vi "update.vi"(8 "error in (no error)":errorcluster, 10 "adapter executability":T1={"instrument"=TRUE, "trajectory"=TRUE, "scanHead"=TRUE, "DAQ"=TRUE, "imageAssembler"=TRUE, "dataCollection"=TRUE, "display"=TRUE, "analyser"=TRUE, "stimulator"=TRUE}, 11 "ScanModeDL090923Scaffold in":refnum<class "ImagingModeDL090923Scaffold.lvclass">) -> (0 "error out":errorcluster, 3 "ScanModeDL090923Scaffold out":refnum<class "ImagingModeDL090923Scaffold.lvclass">)   [LabVIEW 2010, in "ImagingModeDL090923Scaffold.lvclass"]
uses:
  ImagingModeDL090923Scaffold.lvclass
  adapter_executability_cluster.ctl
  Instrument/GenericInstrument/GenericInstrument/GenericInstrument.lvclass
  Trajectory/GenericTrajectory/GenericTrajectory/GenericTrajectory.lvclass
  ScanHead/GenericScanHead/GenericScanHead/GenericScanHead.lvclass
  Stimulator/GenericStimulator/GenericStimulator/GenericStimulator.lvclass
  Analyser/GenericAnalyser/GenericAnalyser/GenericAnalyser.lvclass
  DataCollection/GenericDataCollection/GenericDataCollection/GenericDataCollection.lvclass
  Display/GenericDisplay/GenericDisplay/GenericDisplay.lvclass
  ImageAssembler/GenericImageAssembler/GenericImageAssembler/GenericImageAssembler.lvclass
  DAQ/GenericDAQ/GenericDAQ/GenericDAQ.lvclass
  common/classes/GenericComponent/GenericComponent/GenericComponent.lvclass
  GenericImagingMode/GenericImagingMode/GenericImagingMode.lvclass
  Adapter/GenericAdapter/GenericAdapter/GenericAdapter.lvclass
  common/classes/ErrorController/ErrorController/class_data.vi
  common/classes/ErrorController/ErrorController/ErrorController.lvclass
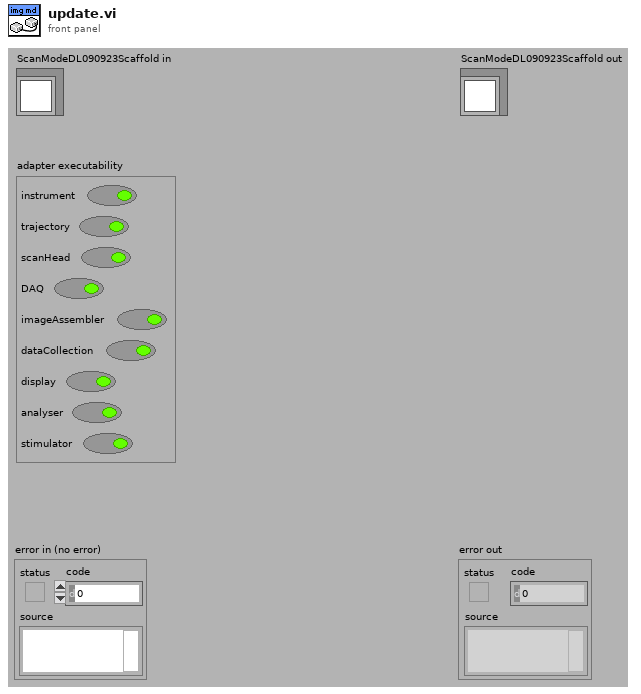
[diagram p1: front panel]
types:
  T1 = typedef "ImagingModeDL090923Scaffold.lvclass/adapter_executability_cluster.ctl" = cluster{"instrument":bool, "trajectory":bool, "scanHead":bool, "DAQ":bool, "imageAssembler":bool, "dataCollection":bool, "display":bool, "analyser":bool, "stimulator":bool}
  T2 = cluster{"[0]":refnum<class "GenericComponent.lvclass">, "[1]":refnum<class "GenericComponent.lvclass">, "[2]":refnum<class "GenericComponent.lvclass">, "[3]":refnum<class "GenericComponent.lvclass">, "[4]":refnum<class "GenericComponent.lvclass">, "[5]":refnum<class "GenericComponent.lvclass">, "[6]":refnum<class "GenericComponent.lvclass">, "[7]":refnum<class "GenericComponent.lvclass">, "[8]":refnum<class "GenericComponent.lvclass">}
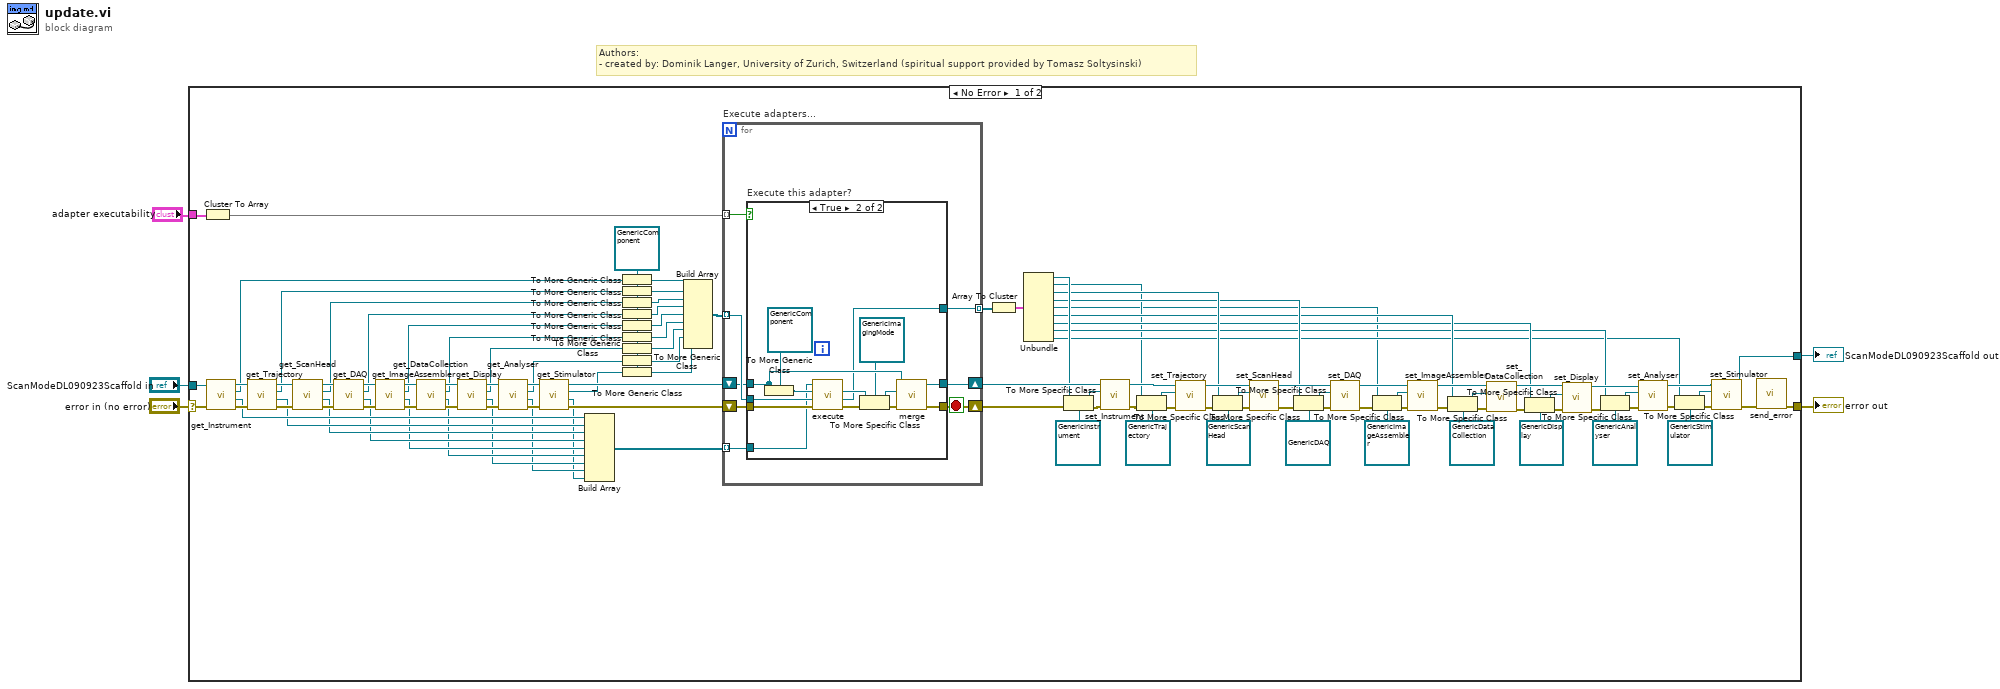
[diagram p0: block diagram]
diagram:
  # "Authors: \n- created by: Dominik Langer, University of Zurich, Switzerland (spiritual support provided by Tomasz Soltysinski)"
  n1 = case shown="No Error" "error in (no error)" {
    selector: "error in (no error)" -> [w76 w142]
    tunnel: [w27 w143] -> w2
    tunnel: "ScanModeDL090923Scaffold in" -> [w9 w143]
    tunnel: [w12 w142] -> w3
    tunnel: "adapter executability" -> [w7 _]
    frame No Error {
      w10 = refnum<class "GenericComponent.lvclass"> refnum ("GenericComponent.lvclass")
      n2 = Cluster To Array(cluster=w7) -> (array=w6:bool[])
      n3 = call-dynamic "get_Instrument.vi"("error in (no error)"=w76, "ScanModeDL090923Scaffold in"=w9) -> ("error out"=w84:errorcluster, "Instrument adapter"=w65:refnum<class "GenericAdapter.lvclass">, "Instrument"=w56:refnum<class "GenericInstrument.lvclass">, "ScanModeDL090923Scaffold out"=w74:refnum<class "ImagingModeDL090923Scaffold.lvclass">)  [unwired: 4 in, 2 out]
      n4 = call-dynamic "get_Trajectory.vi"("error in (no error)"=w84, "ScanModeDL090923Scaffold in"=w74) -> ("error out"=w83:errorcluster, "Trajectory adapter"=w64:refnum<class "GenericAdapter.lvclass">, "Trajectory"=w55:refnum<class "GenericTrajectory.lvclass">, "ScanModeDL090923Scaffold out"=w73:refnum<class "ImagingModeDL090923Scaffold.lvclass">)  [unwired: 2 in, 4 out]
      n5 = call-dynamic "get_ScanHead.vi"("error in (no error)"=w83, "ScanModeDL090923Scaffold in"=w73) -> ("error out"=w82:errorcluster, "ScanHead adapter"=w63:refnum<class "GenericAdapter.lvclass">, "ScanHead"=w54:refnum<class "GenericScanHead.lvclass">, "ScanModeDL090923Scaffold out"=w72:refnum<class "ImagingModeDL090923Scaffold.lvclass">)  [unwired: 4 in, 2 out]
      n6 = call-dynamic "get_DAQ.vi"("error in (no error)"=w82, "ScanModeDL090923Scaffold in"=w72) -> ("error out"=w81:errorcluster, "DAQ adapter"=w62:refnum<class "GenericAdapter.lvclass">, "DAQ"=w53:refnum<class "GenericDAQ.lvclass">, "ScanModeDL090923Scaffold out"=w71:refnum<class "ImagingModeDL090923Scaffold.lvclass">)  [unwired: 4 in, 2 out]
      n7 = call-dynamic "get_ImageAssembler.vi"("error in (no error)"=w81, "ScanModeDL090923Scaffold in"=w71) -> ("error out"=w80:errorcluster, "ImageAssembler adapter"=w61:refnum<class "GenericAdapter.lvclass">, "ImageAssembler"=w52:refnum<class "GenericImageAssembler.lvclass">, "ScanModeDL090923Scaffold out"=w70:refnum<class "ImagingModeDL090923Scaffold.lvclass">)  [unwired: 4 in, 2 out]
      n8 = call-dynamic "get_DataCollection.vi"("error in (no error)"=w80, "ScanModeDL090923Scaffold in"=w70) -> ("error out"=w79:errorcluster, "DataCollection adapter"=w60:refnum<class "GenericAdapter.lvclass">, "DataCollection"=w51:refnum<class "GenericDataCollection.lvclass">, "ScanModeDL090923Scaffold out"=w69:refnum<class "ImagingModeDL090923Scaffold.lvclass">)  [unwired: 4 in, 2 out]
      n9 = call-dynamic "get_Display.vi"("error in (no error)"=w79, "ScanModeDL090923Scaffold in"=w69) -> ("error out"=w78:errorcluster, "Display adapter"=w59:refnum<class "GenericAdapter.lvclass">, "Display"=w50:refnum<class "GenericDisplay.lvclass">, "ScanModeDL090923Scaffold out"=w68:refnum<class "ImagingModeDL090923Scaffold.lvclass">)  [unwired: 4 in, 2 out]
      n10 = call-dynamic "get_Analyser.vi"("error in (no error)"=w78, "ScanModeDL090923Scaffold in"=w68) -> ("error out"=w77:errorcluster, "Analyser adapter"=w58:refnum<class "GenericAdapter.lvclass">, "Analyser"=w49:refnum<class "GenericAnalyser.lvclass">, "ScanModeDL090923Scaffold out"=w67:refnum<class "ImagingModeDL090923Scaffold.lvclass">)  [unwired: 4 in, 2 out]
      n11 = call-dynamic "get_Stimulator.vi"("error in (no error)"=w77, "ScanModeDL090923Scaffold in"=w67) -> ("error out"=w75:errorcluster, "Stimulator adapter"=w57:refnum<class "GenericAdapter.lvclass">, "Stimulator"=w48:refnum<class "GenericStimulator.lvclass">, "ScanModeDL090923Scaffold out"=w66:refnum<class "ImagingModeDL090923Scaffold.lvclass">)  [unwired: 4 in, 2 out]
      n12 = Build Array(w65, w64, w63, w62, w61, w60, w59, w58, w57) -> (w116:refnum<class "GenericAdapter.lvclass">[])
      n13 = To More Generic Class(target class=w10, reference=w56) -> (generic class reference=w115:refnum<class "GenericComponent.lvclass">)
      n14 = To More Generic Class(target class=w10, reference=w55) -> (generic class reference=w113:refnum<class "GenericComponent.lvclass">)
      n15 = To More Generic Class(target class=w10, reference=w54) -> (generic class reference=w112:refnum<class "GenericComponent.lvclass">)
      n16 = To More Generic Class(target class=w10, reference=w53) -> (generic class reference=w111:refnum<class "GenericComponent.lvclass">)
      n17 = To More Generic Class(target class=w10, reference=w52) -> (generic class reference=w110:refnum<class "GenericComponent.lvclass">)
      n18 = To More Generic Class(target class=w10, reference=w51) -> (generic class reference=w109:refnum<class "GenericComponent.lvclass">)
      n19 = To More Generic Class(target class=w10, reference=w50) -> (generic class reference=w114:refnum<class "GenericComponent.lvclass">)
      n20 = To More Generic Class(target class=w10, reference=w49) -> (generic class reference=w101:refnum<class "GenericComponent.lvclass">)
      n21 = To More Generic Class(target class=w10, reference=w48) -> (generic class reference=w99:refnum<class "GenericComponent.lvclass">)
      n22 = Build Array(w115, w113, w112, w111, w110, w109, w114, w101, w99) -> (w108:refnum<class "GenericComponent.lvclass">[])
      n23 = for "Execute adapters..." {
        shift-right: [w118] -> w38
        shift-left: w75 -> [w124]
        tunnel: w116 -> [w119] mode=indexing
        shift-right: [w122] -> w35
        shift-left: w66 -> [w121]
        tunnel: w108 -> [w123] mode=indexing
        tunnel: [w120] -> w8 mode=indexing
        tunnel: w6 -> [w117] mode=indexing
        stop <- w118 stop-if-true
        n24 = case "Execute this adapter?" shown="True" w117 {
          tunnel: w124 -> [w126 w137]
          tunnel: w123 -> [w125 w136]
          tunnel: [w127 w134] -> w122
          tunnel: w121 -> [w127 w133]
          tunnel: [w125 w130] -> w120
          tunnel: w119 -> [_ w129]
          tunnel: [w126 w128] -> w118
          frame False {
          }
          frame True {
            n25 = To More Generic Class(target class=refnum<class "GenericComponent.lvclass"> refnum ("GenericComponent.lvclass"), reference=w133) -> (generic class reference=w138:refnum<class "GenericComponent.lvclass">)
            n26 = call-dynamic "execute.vi"("error in (no error)"=w137, "B in"=w136, "A in"=w138, "GenericAdapter in"=w129) -> ("error out"=w139:errorcluster, "B out"=w130:refnum<class "GenericComponent.lvclass">, "A out"=w140:refnum<class "GenericComponent.lvclass">)  [unwired: 5 out]
            n27 = To More Specific Class(target class=refnum<class "GenericImagingMode.lvclass"> refnum ("GenericImagingMode.lvclass"), reference=w140, error in=w139) -> (specific class reference=w131:refnum<class "GenericImagingMode.lvclass">, error out=w135:errorcluster)
            n28 = call-dynamic "merge.vi"("error in (no error)"=w135, "update"=w131, "GenericScanMode in"=w133) -> ("error out"=w128:errorcluster, "GenericScanMode out"=w134:refnum<class "ImagingModeDL090923Scaffold.lvclass">)  [unwired: 7 in]
          }
        }
      }
      n29 = Array To Cluster(array=w8) -> (cluster=w107:T2)
      n30 = Unbundle(w107) -> ("[0]"=w25:refnum<class "GenericComponent.lvclass">, "[1]"=w17:refnum<class "GenericComponent.lvclass">, "[2]"=w24:refnum<class "GenericComponent.lvclass">, "[3]"=w23:refnum<class "GenericComponent.lvclass">, "[4]"=w14:refnum<class "GenericComponent.lvclass">, "[5]"=w22:refnum<class "GenericComponent.lvclass">, "[6]"=w21:refnum<class "GenericComponent.lvclass">, "[7]"=w20:refnum<class "GenericComponent.lvclass">, "[8]"=w19:refnum<class "GenericComponent.lvclass">)
      n31 = To More Specific Class(target class=refnum<class "GenericInstrument.lvclass"> refnum ("GenericInstrument.lvclass"), reference=w25, error in=w38) -> (specific class reference=w85:refnum<class "GenericInstrument.lvclass">, error out=w45:errorcluster)
      n32 = call-dynamic "set_Instrument.vi"("error in (no error)"=w45, "GenericInstrument.lvclass"=w85, "ScanModeDL090923Scaffold in"=w35) -> ("error out"=w44:errorcluster, "ScanModeDL090923Scaffold out"=w34:refnum<class "ImagingModeDL090923Scaffold.lvclass">)  [unwired: 7 in]
      n33 = To More Specific Class(target class=refnum<class "GenericTrajectory.lvclass"> refnum ("GenericTrajectory.lvclass"), reference=w17, error in=w44) -> (specific class reference=w87:refnum<class "GenericTrajectory.lvclass">, error out=w43:errorcluster)
      n34 = call-dynamic "set_Trajectory.vi"("error in (no error)"=w43, "GenericTrajectory.lvclass"=w87, "ScanModeDL090923Scaffold in"=w34) -> ("error out"=w42:errorcluster, "ScanModeDL090923Scaffold out"=w33:refnum<class "ImagingModeDL090923Scaffold.lvclass">)  [unwired: 7 in]
      n35 = To More Specific Class(target class=refnum<class "GenericScanHead.lvclass"> refnum ("GenericScanHead.lvclass"), reference=w24, error in=w42) -> (specific class reference=w90:refnum<class "GenericScanHead.lvclass">, error out=w91:errorcluster)
      n36 = call-dynamic "set_ScanHead.vi"("error in (no error)"=w91, "GenericScanHead.lvclass"=w90, "ScanModeDL090923Scaffold in"=w33) -> ("error out"=w39:errorcluster, "ScanModeDL090923Scaffold out"=w32:refnum<class "ImagingModeDL090923Scaffold.lvclass">)  [unwired: 7 in]
      n37 = To More Specific Class(target class=refnum<class "GenericDAQ.lvclass"> refnum ("GenericDAQ.lvclass"), reference=w23, error in=w39) -> (specific class reference=w98:refnum<class "GenericDAQ.lvclass">, error out=w40:errorcluster)
      n38 = call-dynamic "set_DAQ.vi"("error in (no error)"=w40, "GenericDAQ.lvclass"=w98, "ScanModeDL090923Scaffold in"=w32) -> ("error out"=w16:errorcluster, "ScanModeDL090923Scaffold out"=w15:refnum<class "ImagingModeDL090923Scaffold.lvclass">)  [unwired: 7 in]
      n39 = To More Specific Class(target class=refnum<class "GenericImageAssembler.lvclass"> refnum ("GenericImageAssembler.lvclass"), reference=w14, error in=w16) -> (specific class reference=w18:refnum<class "GenericImageAssembler.lvclass">, error out=w11:errorcluster)
      n40 = call-dynamic "set_ImageAssembler.vi"("error in (no error)"=w11, "GenericImageAssembler.lvclass"=w18, "ScanModeDL090923Scaffold in"=w15) -> ("error out"=w37:errorcluster, "ScanModeDL090923Scaffold out"=w31:refnum<class "ImagingModeDL090923Scaffold.lvclass">)  [unwired: 7 in]
      n41 = To More Specific Class(target class=refnum<class "GenericDataCollection.lvclass"> refnum ("GenericDataCollection.lvclass"), reference=w22, error in=w37) -> (specific class reference=w94:refnum<class "GenericDataCollection.lvclass">, error out=w95:errorcluster)
      n42 = call-dynamic "set_DataCollection.vi"("error in (no error)"=w95, "GenericDataCollection.lvclass"=w94, "ScanModeDL090923Scaffold in"=w31) -> ("error out"=w26:errorcluster, "ScanModeDL090923Scaffold out"=w30:refnum<class "ImagingModeDL090923Scaffold.lvclass">)  [unwired: 7 in]
      n43 = To More Specific Class(target class=refnum<class "GenericDisplay.lvclass"> refnum ("GenericDisplay.lvclass"), reference=w21, error in=w26) -> (specific class reference=w96:refnum<class "GenericDisplay.lvclass">, error out=w97:errorcluster)
      n44 = call-dynamic "set_Display.vi"("error in (no error)"=w97, "GenericDisplay.lvclass"=w96, "ScanModeDL090923Scaffold in"=w30) -> ("error out"=w36:errorcluster, "ScanModeDL090923Scaffold out"=w29:refnum<class "ImagingModeDL090923Scaffold.lvclass">)  [unwired: 7 in]
      n45 = To More Specific Class(target class=refnum<class "GenericAnalyser.lvclass"> refnum ("GeneralAnalyser.lvclass"), reference=w20, error in=w36) -> (specific class reference=w92:refnum<class "GenericAnalyser.lvclass">, error out=w93:errorcluster)
      n46 = call-dynamic "set_Analyser.vi"("error in (no error)"=w93, "Analyser"=w92, "ScanModeDL090923Scaffold in"=w29) -> ("error out"=w41:errorcluster, "ScanModeDL090923Scaffold out"=w28:refnum<class "ImagingModeDL090923Scaffold.lvclass">)  [unwired: 7 in]
      n47 = To More Specific Class(target class=refnum<class "GenericStimulator.lvclass"> refnum ("GenericStimulator.lvclass"), reference=w19, error in=w41) -> (specific class reference=w88:refnum<class "GenericStimulator.lvclass">, error out=w89:errorcluster)
      n48 = call-dynamic "set_Stimulator.vi"("error in (no error)"=w89, "GenericStimulator.lvclass"=w88, "ScanModeDL090923Scaffold in"=w28) -> ("error out"=w13:errorcluster, "ScanModeDL090923Scaffold out"=w27:refnum<class "ImagingModeDL090923Scaffold.lvclass">)  [unwired: 7 in]
      n49 = call "send_error.vi"("error in (no error)"=w13) -> ("error out"=w12:errorcluster)  [unwired: 10 in]
    }
    frame Error {
    }
  }
  "error out" <- w3
  "ScanModeDL090923Scaffold out" <- w2
